vi "test -- PLL analyzer -- V2.vi"() -> ()   [LabVIEW 2017]
uses:
  lorentzian.ctl
  circle corners.ctl
  pid -- parameters.ctl
  <vilib>/event_ctls.llb/eventvkey.ctl
  cursor winow.ctl
  show-win- control.ctl
  PID action.ctl
  cursor window action.ctl
  agregator -- action.ctl
  interpolation state - real.ctl
  publisher action.ctl
  four-corner circle transformation.ctl
  cursor action.ctl
  linear interpolation - real.vi
  draw a line.vi
  draw a circle.vi
  linear interpolation iiii- complex.vi
  Q - not nan -- real.vi
  generate linear region.vi
panel:
  in  "all 3":enum32{"all", "other"}(tab)
  in  "reset freq":bool
  in  "dt (sec)":dbl=0.001 format="%#_10f"
  out "Plot: complex plane - filter":cluster{dbl[], dbl[]}[](graph)=[{[0.00032340920609960806, 0.00032267756333283855, 0.0003204839185825568, 0.0003168321202470601, 0.00031172857482151867, 0.00030518223565880506, 0.0002972045872622716, 0.0002878096251380292, 0.0002770138312420732, 0.00026483614506533264, 0.00025129793040736686, 0.00023642293789700238, 0.00022023726332565878, 0.00020276930186646325, 0.00018404969825946873, 0.00016411129305036554, 0.00014298906497700625, 0.00012072006960481285, 9.734337431872354e-05, 7.289998978572481e-05, 4.743279800820512e-05, 2.098647709435238e-05, -6.392577122430495e-06, -3.465633247758186e-05, -6.37552047401204e-05, -9.363814460023435e-05, -0.00012425272722711787, -0.0001555452442399381, -0.0001874607979305862, -0.00021994339757291058, -0.00025293605764947704, -0.00028638089782352986, -0.0003202192444807712, -0.00035439173366281644, -0.00038883841521175036, -0.00042349885794307543, -0.0004583122556625431, -0.0004932175338408814, -0.0005281534567592722, -0.0005630587349376105, -0.0005978721326570782, -0.000632532575388403, -0.0006669792569373372, -0.0007011517461193825, -0.0007349900927766238, -0.0007684349329506767, -0.0008014275930272432, -0.0008339101926695676, -0.0008658257463602154, -0.0008971182633730359, -0.0009277328459999193, -0.0009576157858600333, -0.000986714658122572, -0.0010149784134777233, -0.001042357467694506, -0.0010688037886083589, -0.0010942709803858784, -0.0011187143649188773, -0.0011420910602049665, -0.0011643600555771602, -0.0011854822836505194, -0.0012054206888596224, -0.0012241402924666172, -0.0012416082539258126, -0.0012577939284971562, -0.0012726689210075207, -0.0012862071356654864, -0.0012983848218422272, -0.0013091806157381832, -0.0013185755778624254, -0.001326553226258959, -0.0013330995654216725, -0.001338203110847214, -0.0013418549091827109, -0.0013440485539329924, -0.001344780196699762, -0.0013440485539329924, -0.0013418549091827109, -0.001338203110847214, -0.0013330995654216725, -0.001326553226258959, -0.0013185755778624257, -0.0013091806157381832, -0.0012983848218422272, -0.0012862071356654866, -0.001272668921007521, -0.0012577939284971564, -0.0012416082539258128, -0.0012241402924666174, -0.001205420688859623, -0.0011854822836505196, -0.0011643600555771604, -0.001142091060204967, -0.0011187143649188777, -0.0010942709803858789, -0.0010688037886083593, -0.0010423574676945067, -0.001014978413477724, -0.0009867146581225724, -0.0009576157858600338, -0.0009277328459999199, -0.0008971182633730364, -0.0008658257463602159, -0.0008339101926695678, -0.0008014275930272436, -0.000768434932950677, -0.000734990092776624, -0.0007011517461193834, -0.0006669792569373381, -0.000632532575388404, -0.000597872132657079, -0.0005630587349376113, -0.0005281534567592729, -0.000493217533840882, -0.0004583122556625437, -0.00042349885794307603, -0.0003888384152117509, -0.0003543917336628168, -0.00032021924448077157, -0.00028638089782353024, -0.0002529360576494772, -0.00021994339757291145, -0.00018746079793058703, -0.00015554524423993897, -0.00012425272722711857, -9.3638144600235e-05, -6.375520474012104e-05, -3.4656332477582454e-05, -6.392577122430929e-06, 2.0986477094351945e-05, 4.7432798008204685e-05, 7.289998978572449e-05, 9.734337431872332e-05, 0.00012072006960481252, 0.00014298906497700603, 0.00016411129305036543, 0.00018404969825946808, 0.00020276930186646292, 0.00022023726332565834, 0.00023642293789700205, 0.00025129793040736654, 0.0002648361450653323, 0.000277013831242073, 0.0002878096251380291, 0.0002972045872622715, 0.00030518223565880495, 0.00031172857482151856, 0.0003168321202470601, 0.0003204839185825567, 0.00032267756333283855], [0.00031496097830625033, 0.0003498892391994237, 0.00038475622405428764, 0.00041950076433152565, 0.00045406190630121736, 0.0004883790179763929, 0.0005223918954821412, 0.0005560408686736638, 0.0005892669058179846, 0.0006220117171556694, 0.0006542178571608702, 0.0006858288253202979, 0.0007167891652543217, 0.0007470445620063031, 0.0007765419373294864, 0.0008052295428042793, 0.0008330570506225647, 0.0008599756418797792, 0.0008859380922198584, 0.0009108988546828062, 0.0009348141396095384, 0.0009576419914638252, 0.000979342362436558, 0.0009998771827032147, 0.001019210427211269, 0.0010373081788803734, 0.0010541386881044424, 0.001069672428451252, 0.0010838821484618333, 0.0010967429194587922, 0.0011082321792796812, 0.0011183297718586971, 0.0011270179825872719, 0.0011342815693915135, 0.001140107789471984, 0.001144486421658899, 0.001147409784343534, 0.0011488727489543746, 0.0011488727489543746, 0.001147409784343534, 0.001144486421658899, 0.001140107789471984, 0.0011342815693915135, 0.001127017982587272, 0.0011183297718586971, 0.0011082321792796812, 0.0010967429194587925, 0.0010838821484618333, 0.0010696724284512522, 0.0010541386881044426, 0.0010373081788803734, 0.0010192104272112692, 0.0009998771827032147, 0.000979342362436558, 0.0009576419914638255, 0.0009348141396095387, 0.0009108988546828065, 0.0008859380922198587, 0.0008599756418797793, 0.000833057050622565, 0.0008052295428042794, 0.0007765419373294868, 0.0007470445620063036, 0.000716789165254322, 0.0006858288253202981, 0.0006542178571608704, 0.0006220117171556695, 0.0005892669058179848, 0.0005560408686736642, 0.0005223918954821417, 0.0004883790179763933, 0.00045406190630121763, 0.0004195007643315259, 0.00038475622405428786, 0.00034988923919942387, 0.0003149609783062508, 0.0002800327174130774, 0.0002451657325582134, 0.00021042119228097535, 0.00017586005031128358, 0.00014154293863610795, 0.00010753006113035959, 7.38810879388374e-05, 4.0655050794516443e-05, 7.910239456831666e-06, -2.429590054836919e-05, -5.590686870779693e-05, -8.68672086418208e-05, -0.00011712260539380236, -0.0001466199807169854, -0.00017530758619177826, -0.00020313509401006374, -0.00023005368526727817, -0.00025601613560735756, -0.00028097689807030546, -0.00030489218299703763, -0.0003277200348513243, -0.000349420405824057, -0.0003699552260907138, -0.0003892884705987683, -0.00040738622226787243, -0.0004242167314919416, -0.00043975047183875127, -0.00045396019184933253, -0.0004668209628462916, -0.0004783102226671804, -0.0004884078152461965, -0.0004970960259747711, -0.0005043596127790127, -0.0005101858328594831, -0.0005145644650463984, -0.0005174878277310334, -0.000518950792341874, -0.000518950792341874, -0.0005174878277310334, -0.0005145644650463984, -0.0005101858328594832, -0.0005043596127790129, -0.0004970960259747713, -0.0004884078152461966, -0.0004783102226671805, -0.000466820962846292, -0.00045396019184933286, -0.0004397504718387517, -0.00042421673149194215, -0.000407386222267873, -0.00038928847059876883, -0.00036995522609071434, -0.00034942040582405765, -0.00032772003485132494, -0.00030489218299703817, -0.0002809768980703059, -0.000256016135607358, -0.00023005368526727871, -0.0002031350940100644, -0.0001753075861917788, -0.00014661998071698658, -0.00011712260539380328, -8.686720864182172e-05, -5.590686870779785e-05, -2.429590054837011e-05, 7.910239456830636e-06, 4.065505079451547e-05, 7.388108793883637e-05, 0.00010753006113035894, 0.00014154293863610727, 0.00017586005031128293, 0.00021042119228097467, 0.00024516573255821275, 0.0002800327174130767]}, {[0.00017614197280843374, 0.00010745922599758267, 3.8776479186731605e-05, -2.990626762411946e-05, -9.858901443497053e-05, -0.00016727176124582157, -0.00023595450805667266, -0.00030463725486752375, -0.0003733200016783748, -0.00044200274848922583, -0.0005106854953000769, -0.000579368242110928, -0.000648050988921779, -0.0007167337357326301, -0.0007854164825434812, -0.0008540992293543323, -0.0009227819761651833, -0.0009914647229760344, -0.0010601474697868854, -0.0011288302165977364], [-0.00015830638794107768, -0.00011097965131634489, -6.365291469161208e-05, -1.6326178066879268e-05, 3.100055855785353e-05, 7.832729518258632e-05, 0.00012565403180731915, 0.00017298076843205192, 0.00022030750505678474, 0.00026763424168151756, 0.00031496097830625033, 0.0003622877149309831, 0.000409614451555716, 0.00045694118818044875, 0.0005042679248051815, 0.0005515946614299144, 0.0005989213980546472, 0.0006462481346793799, 0.0006935748713041128, 0.0007409016079288456]}, {[-0.000983952861547405, -0.0009366261249226722, -0.0008892993882979395, -0.0008419726516732066, -0.0007946459150484738, -0.000747319178423741, -0.0006999924417990082, -0.0006526657051742754, -0.0006053389685495426, -0.0005580122319248099, -0.0005106854953000771, -0.0004633587586753442, -0.00041603202205061144, -0.00036870528542587867, -0.0003213785488011458, -0.000274051812176413, -0.00022672507555168025, -0.00017939833892694748, -0.0001320716023022147, -8.474486567748183e-05], [-0.0003718664898022604, -0.00030318374299140934, -0.00023450099618055824, -0.00016581824936970718, -9.713550255885611e-05, -2.8452755748005075e-05, 4.022999106284602e-05, 0.00010891273787369711, 0.00017759548468454815, 0.0002462782314953992, 0.0003149609783062502, 0.00038364372511710137, 0.0004523264719279524, 0.0005210092187388034, 0.0005896919655496546, 0.0006583747123605056, 0.0007270574591713567, 0.0007957402059822077, 0.0008644229527930588, 0.0009331056996039098]}, {[-0.0007703927596862223, -0.0006757392864367567, -0.0005810858131872911, -0.00048643233993782547, -0.0003917788666883599, -0.0002971253934388943, -0.00020247192018942864, -0.0001078184469399631, -1.316497369049745e-05, 8.14884995589682e-05, 0.00017614197280843374, 0.0002707954460578993, 0.00036544891930736503, 0.00046010239255683057, 0.0005547558658062961, 0.0006494093390557619, 0.0007440628123052274, 0.0008387162855546929, 0.0009333697588041587, 0.0010280232320536242], [-0.001531961324158099, -0.001394595830536397, -0.0012572303369146947, -0.0011198648432929927, -0.0009824993496712906, -0.0008451338560495885, -0.0007077683624278863, -0.0005704028688061841, -0.00043303737518448206, -0.00029567188156278, -0.0001583063879410779, -2.0940894319375607e-05, 0.00011642459930232647, 0.00025379009292402855, 0.00039115558654573084, 0.0005285210801674329, 0.000665886573789135, 0.0008032520674108371, 0.0009406175610325391, 0.0010779830546542412]}]
  in  "PID parameters":T1={"P (sec)"=1.2701010101010102, "I (sec)"=0.7070707070707071}
  in  "visc hist time (sec)":dbl=15.0 format="%#_10f"
  in  "I (sec)":dbl(slide)=0.7070707070707071 scale=0.0..10.0
  in  "P (sec)":dbl(slide)=1.2701010101010102 scale=0.01..5.0
  in  "circle lorentzian":T2={"Amplitude"=0.002770252259498593, "omega(0)"=44853.30628564185, "Gamma"=3.3212682622846827, "phase"=4.109041090077058, "Q"=13504.87306158988, "Norm  Ampl"=nan, "z (inf)"=0.00017614197280843374-0.00015830638794107763i, "4corners"={"z (-pi/2)"=-0.0009839528615474048-0.0003718664898022611i, "z(inf)"=0.00017614197280843374-0.00015830638794107763i, "z (pi/2)"=-3.741812905274977e-05+0.001001788446414761i, "z center"=-0.0005106854953000773+0.00031496097830624995i, "z(0)"=-0.0011975129634085883+0.0007882283445535775i, "radius"=0.0008340947013996851}} {"z (inf)" format="%#9_9f"; "Q" format="%#9_9f"; "phase" format="%#9_9f"; "Gamma" format="%#9_9f"; "omega(0)" format="%#9_9f"}
  in  "time int ave time (sec)":dbl=0.05 format="%#_10f"
  in  "reset lor":bool
  in  "get fit!":bool
  in  "PLL away!":bool
  in  "PLL limits":dbl=5000.0 format="%#.2f"
  out "zi freq":dbl=44852.18508129662 format="%#.4f"
  out "off freq":dbl=1.1212043452251237 format="%#.8f"
  in  "cursor bracket: fit boundaries":T4={"left"=1.25, "right "=3.75, "center"=2.5, "window"=2.5, "cursors"=[0, 1, 2], "relative"=0, "absolute"=0, "fixed vertical offset"=0.0, "vertical offset"=0.0, "skew"=0.0, "default window frac"=0.1, "kind"=enum."symmetric", "skew.left"=0.5, "skew.right"=0.5, "Plot ref"=refnum, "wing order"=enum."forw"}
  out "VKey":T5
  out "Char":i16=49
  in  "lorentzian -- basic":T2={"Amplitude"=1.0, "omega(0)"=1000.0, "Gamma"=3.0, "phase"=0.0, "Q"=300.0, "Norm  Ampl"=nan, "z (inf)"=0.0+0.0i, "4corners"={"z (-pi/2)"=9.277908004825974e-07+0.0007240755403629966i, "z(inf)"=2.6527949823343002e-05+0.0007477540585896028i, "z (pi/2)"=2.8494315967368497e-06+0.0007733542176124632i, "z center"=1.8886111986097237e-06+0.0007487148789877299i, "z(0)"=-2.2750727426123552e-05+0.000749675699385857i, "radius"=2.4658065287076567e-05}} {"z (inf)" format="%#9_9f"; "Q" format="%#9_9f"; "phase" format="%#9_9f"; "Gamma" format="%#9_9f"; "omega(0)" format="%#9_9f"}
  out "DO reset freq !":bool
  in  "all":enum32{"all", "other"}(tab)
  in  "send for fit!":bool=TRUE
  out "Plot: complex- hist":cluster{dbl[], dbl[]}[](graph)
  out "Plot: hist":cluster{"all rows":dbl[], "all rows":dbl[]}[](graph)
  out "dev freq":dbl=44853.30628564185 format="%#.2f"
  out "win":T6={"center freq (Hz)"=-0.35260838541595674, "window  (Hz)"=17.234446484426172, "left freq (Hz)"=-8.969831627629043, "right freq (Hz)"=8.26461485679713}
  out "zi freq temporary":dbl=44852.18508134297 format="%#.2f"
  out "freq out":dbl[](array[numeric])
  out "v out":cdb[](array[numeric])
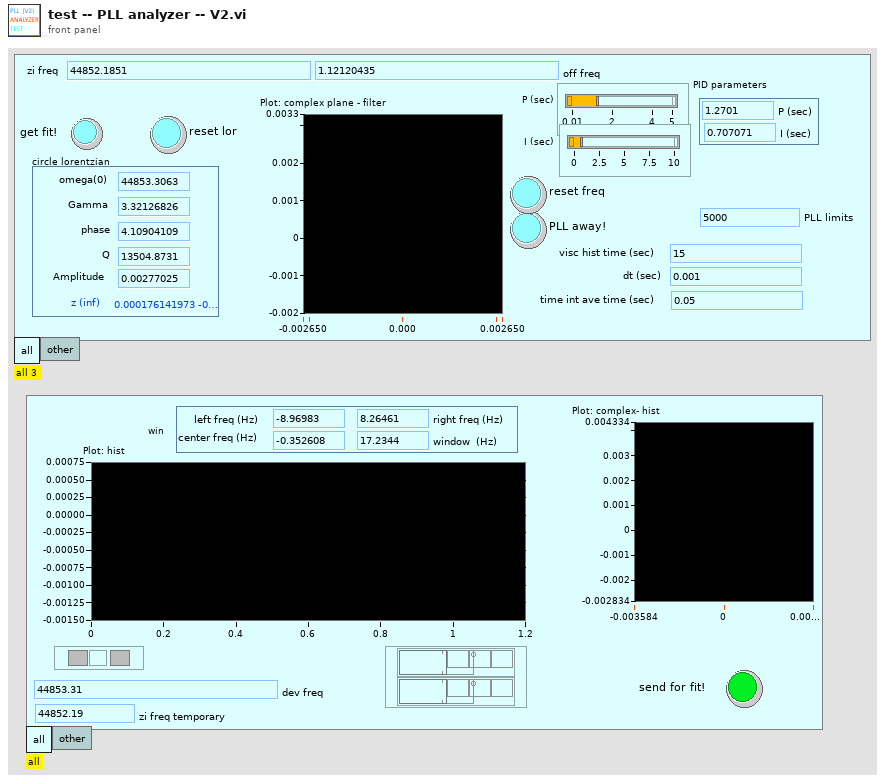
[diagram p1: front panel]
types:
  T1 = typedef "pid -- parameters.ctl" = cluster{"P (sec)":dbl, "I (sec)":dbl}
  T2 = typedef "lorentzian.ctl" = cluster{"Amplitude":dbl, "omega(0)":dbl, "Gamma":dbl, "phase":dbl, "Q":dbl, "Norm  Ampl":dbl, "z (inf)":cdb, "4corners":T3}
  T3 = typedef "circle corners.ctl" = cluster{"z (-pi/2)":cdb, "z(inf)":cdb, "z (pi/2)":cdb, "z center":cdb, "z(0)":cdb, "radius":dbl}
  T4 = typedef "cursor winow.ctl" = cluster{"left":dbl, "right ":dbl, "center":dbl, "window":dbl, "cursors":i32[], "relative":i32, "absolute":i32, "fixed vertical offset":dbl, "vertical offset":dbl, "skew":dbl, "default window frac":dbl, "kind":enum16{"symmetric", "skewed", "fancy"}, "skew.left":dbl, "skew.right":dbl, "Plot ref":refnum<vi>, "wing order":enum16{"forw", "back"}}
  T5 = typedef "eventvkey.ctl" = enum16{"ASCII", "Enter", "Return", "Shift", "Ctrl", "Alt", "Cmd", "Opt", "Caps", "NumLock", "Clear", "Break", "Up", "Down", "Left", "Right", "Insert", "Delete", "Home", "End", "PageUp", "PageDown", "Escape", "Help", "Pause", "ScrollLock", "F1", "F2", "F3", "F4", "F5", "F6", "F7", "F8", "F9", "F10", "F11", "F12", "F13", "F14", "F15", "F16", "F17", "F18", "F19", "F20", "F21", "F22", "F23", "F24", "Play", "VolumeUp", "VolumeDown", "Mute", "Two Byte Char"}
  T6 = typedef "show-win- control.ctl" = cluster{"center freq (Hz)":dbl, "window  (Hz)":dbl, "left freq (Hz)":dbl, "right freq (Hz)":dbl}
  T7 = typedef "publisher action.ctl" = enum16{"set", "get"}
  T8 = typedef "interpolation state - real.ctl" = cluster{"requested size":i32, "Array":dbl[], "actual number of elements":i32}
  T9 = typedef "agregator -- action.ctl" = enum16{"append", "interpolate", "empty!", "force", "init", "scale", "read last"}
  T10 = typedef "cursor window action.ctl" = enum16{"balance", "h. offset change", "cursor moves", "change center", "change window", "init", "check", "reset", "set y to middle", "idle", "-write all Y", "-write left.X", "-write center.X", "-write right.X", "-write all X", "-change center", "-change window", "-change skew", "-read cursor 2", "-read cursor 1", "-read cursor 0", "-read all cursors", "-reset", "-read plot scale", "-set y to middle", "-Q: center.Y is visible", "-Q: window is visible", "-parse center.Y", "-right left from center", "-left move", "-right move", "-set center.Y", "-empty", "-set cursors to default", "-check", "-write center.Y", "-copy cursor 1", "-copy cursor 0", "-copy cursor 2", "move right", "move left", "shrink", "broaden", "skew up", "skew down", "-write plot scale", "zoom X", "change cen&win", "zoom to all data", "color--red", "color--green", "color--yellow", "read", "zoom out", "zoom in", "slide right", "slide left", "set range aspect ratio to 1"}
  T11 = typedef "PID action.ctl" = enum16{"append", "empty!", "reset frequency"}
  T12 = typedef "Zurich Instruments LabOne.lvlib/ziTypeHandle.ctl" = cluster{"handleValid":bool, "Conn":u64, "Path Prefix":string, "Handle":u64, "Connected":bool, "Clockbase(s)":dbl}
  T13 = typedef "cursor action.ctl" = enum16{"range", "read", "write", "check", "zoom out", "smart zoom out", "zoom to aspect ratio 1"}
  T14 = typedef "four-corner circle transformation.ctl" = enum16{"z(c) z(inf)", "z(c) z(zero)", "fix phase", "calculate lorentzian", "z(0) z(+-pi/2)", "shift to zcenter", "to  canonical", "get canonical phase", "get4corners"}
  T15 = typedef "interpolation state - complex.ctl" = cluster{"requested size":i32, "Array":cdb[], "actual number of elements":i32}
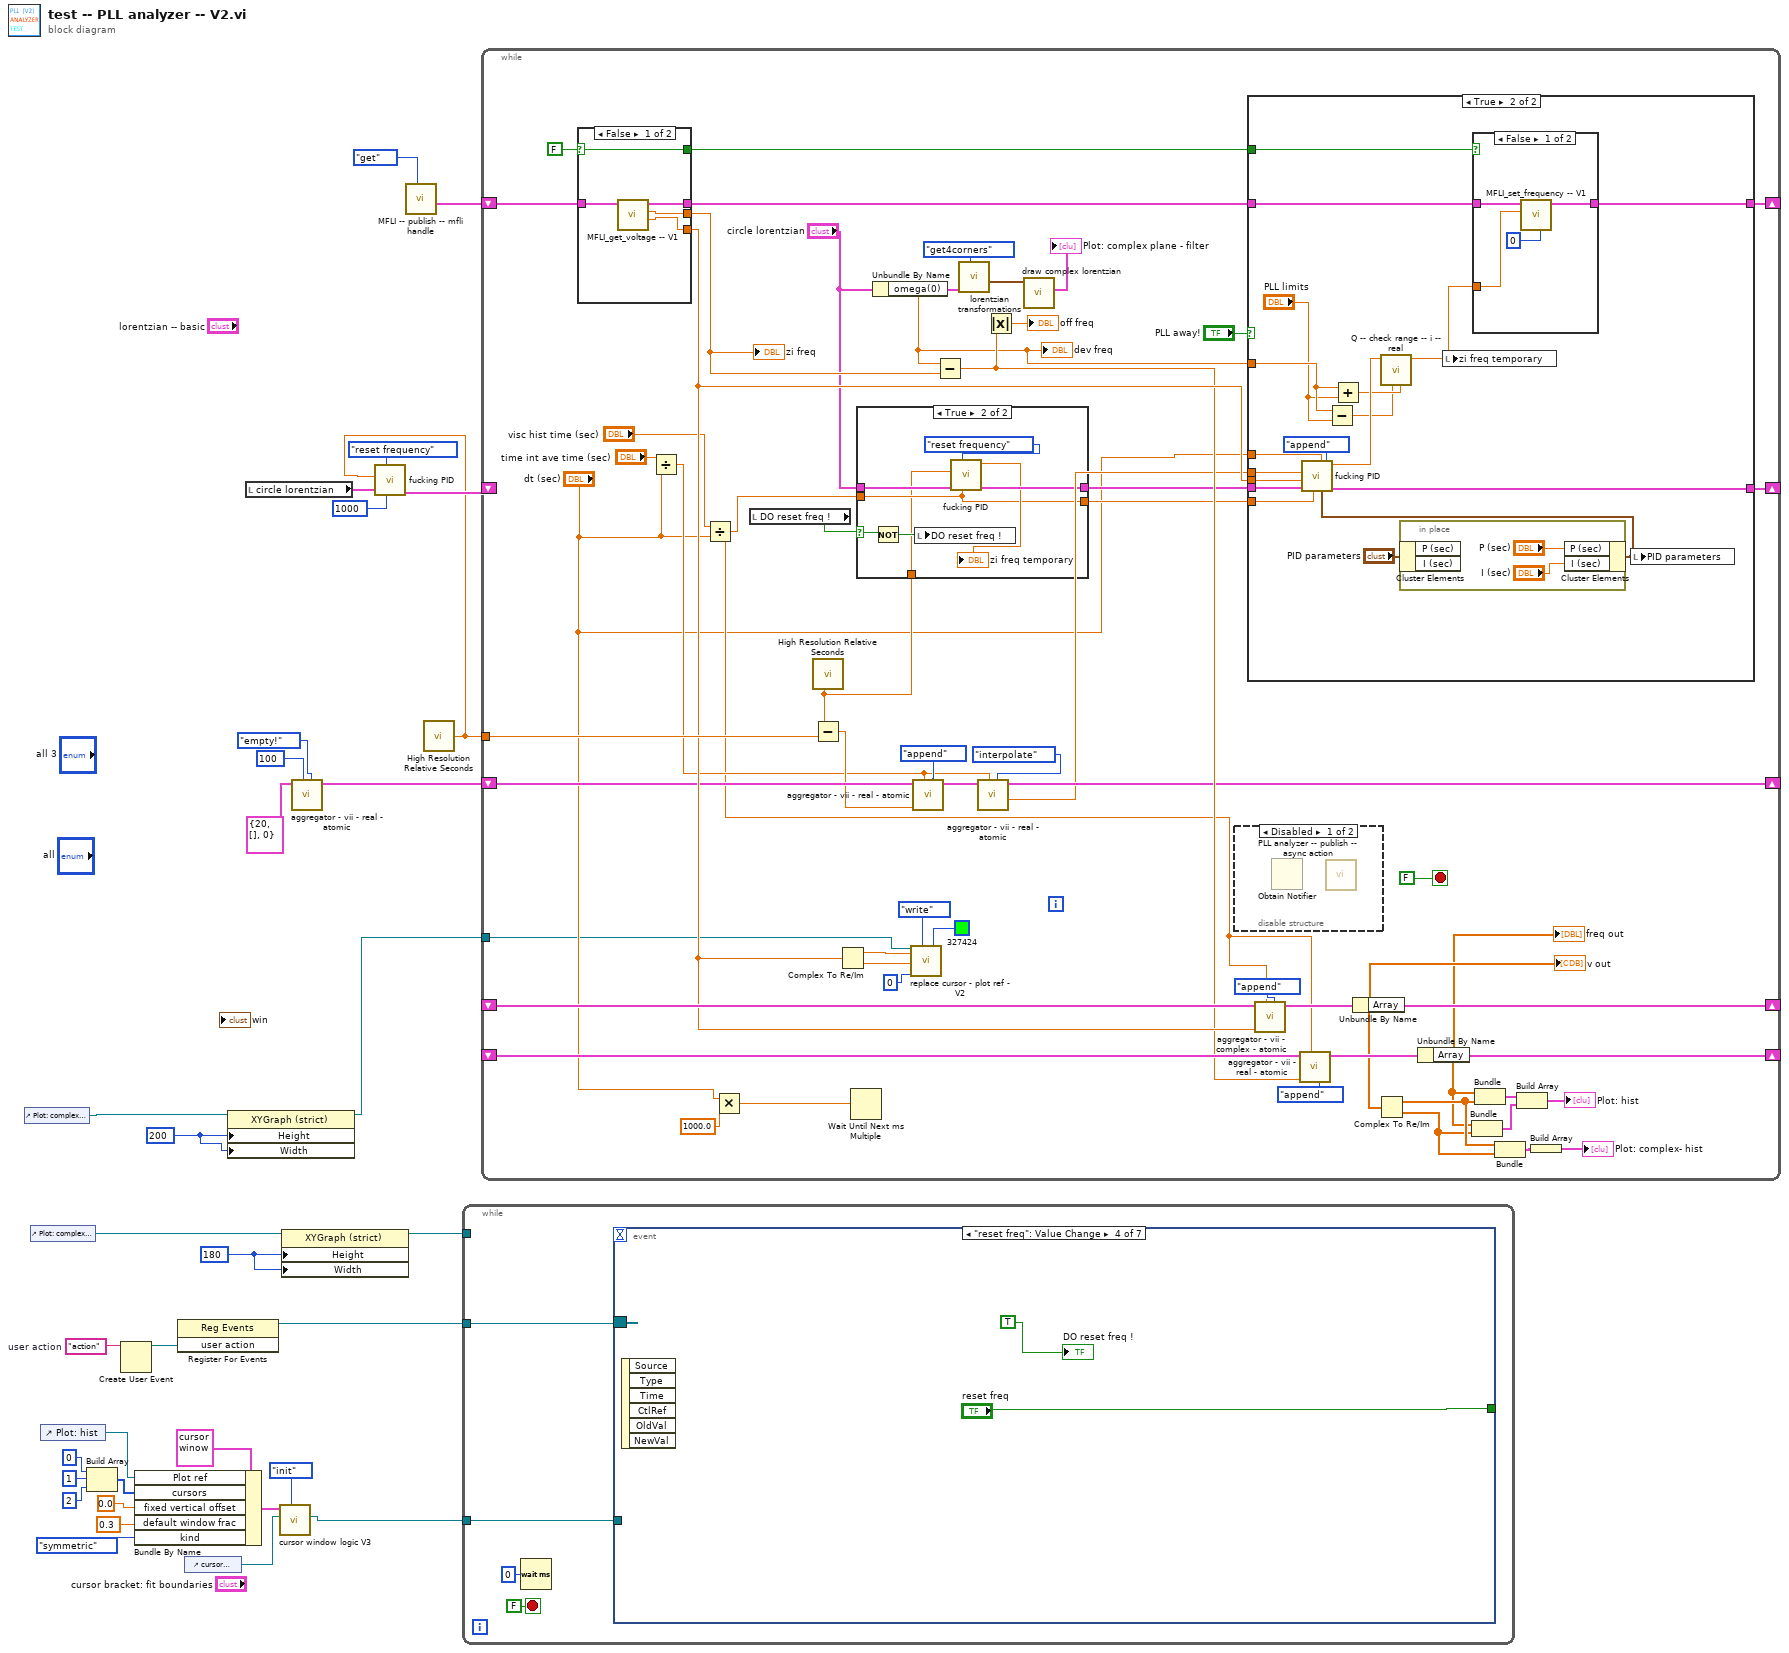
[diagram p0: block diagram]
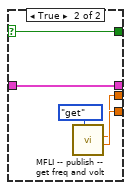
[diagram p2: hidden frame]
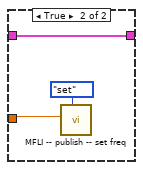
[diagram p4: hidden frame]
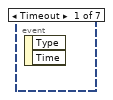
[diagram p7: hidden frame]
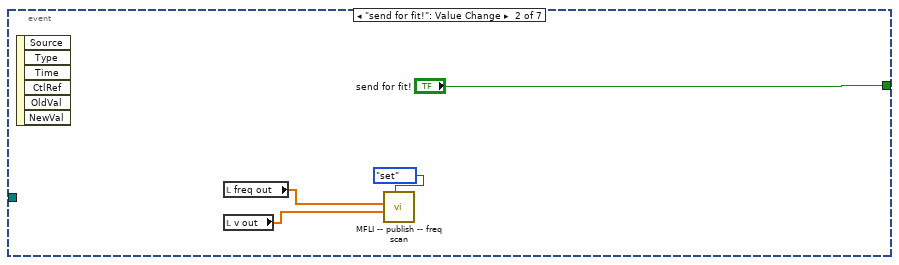
[diagram p8: hidden frame]
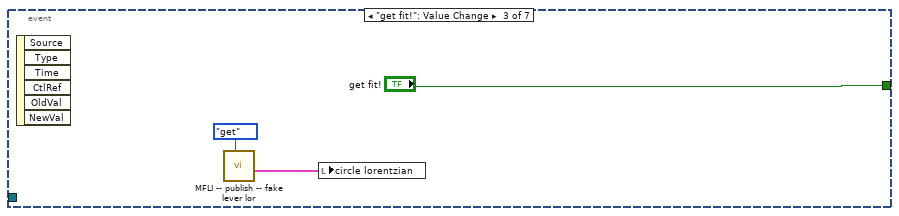
[diagram p9: hidden frame]
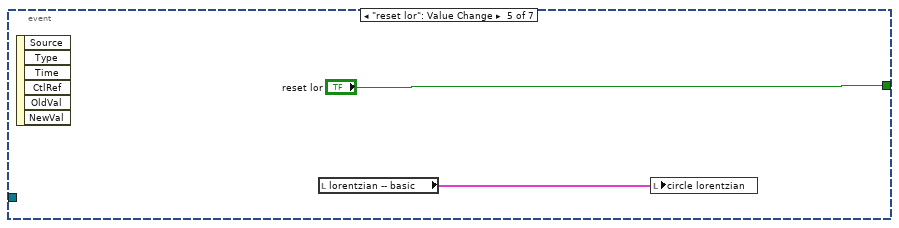
[diagram p10: hidden frame]
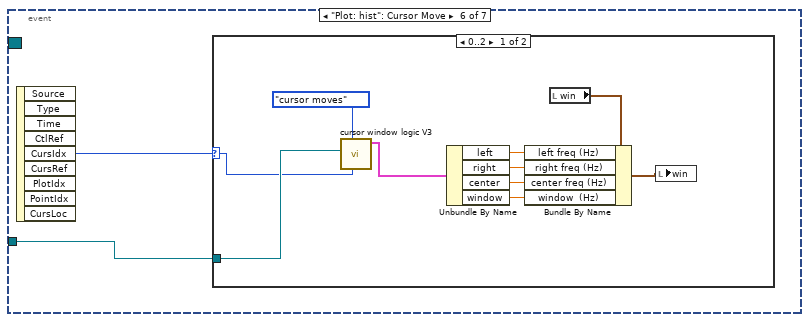
[diagram p11: hidden frame]
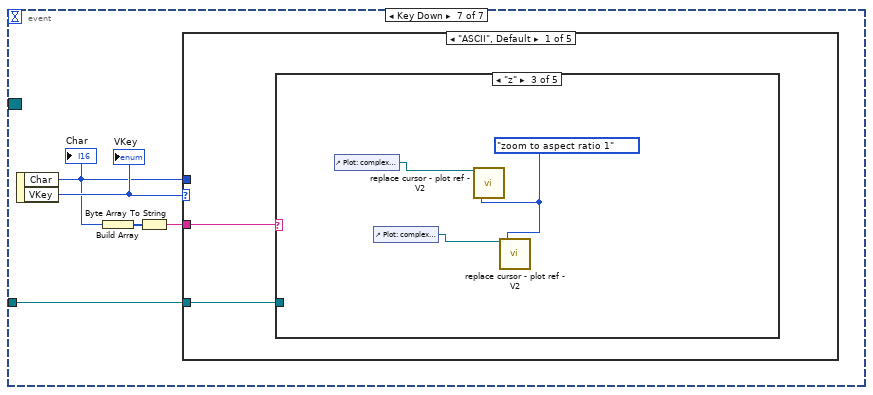
[diagram p13: hidden frame]
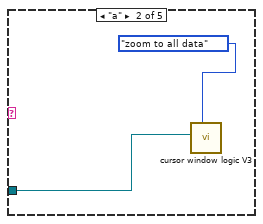
[diagram p15: hidden frame]
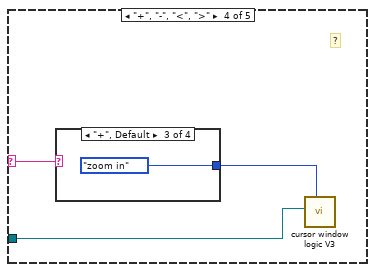
[diagram p16: hidden frame]
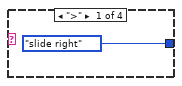
[diagram p17: hidden frame]
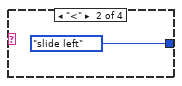
[diagram p18: hidden frame]
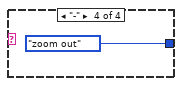
[diagram p19: hidden frame]
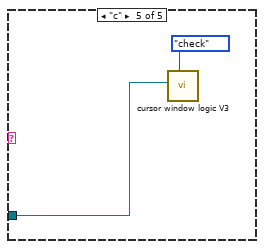
[diagram p20: hidden frame]
diagram:
  w4 = u32 180 ("Plot Area:Size:Height")
  w6 = u32 200 ("Plot Area:Size:Height")
  w30 = "action"  # user action
  n1 = control-ref of="Plot: complex plane - filter"() -> (w7:refnum<vi>)
  n2 = control-ref of="Plot: complex- hist"() -> (w1:refnum<vi>)
  n3 = control-ref of="Plot: hist"() -> (w3:refnum<vi>)
  n4 = Build Array(0, 1, 2) -> (w18:i32[])
  n5 = Create User Event(user event datatype=w30) -> (user event=w31:refnum<user-event>)  [unwired: 1 in, 1 out]
  n6 = Bundle By Name(cluster=T4 {"left"=0.0, "right "=0.0, "center"=0.0, "window"=0.0, "cursors"=[], "relative"=0, "absolute"=0, "fixed vertical offset"=0.0, "vertical offset"=0.0, "skew"=0.0, "default window frac"=0.0, "kind"=enum."symmetric", "skew.left"=0.0, "skew.right"=0.0, "Plot ref"=refnum, "wing order"=enum."forw"} ("cursor bracket: All, data window"), "Plot ref"=w3, "cursors"=w18, "fixed vertical offset"=0.0, "default window frac"=0.3 ("fixed vertical offset"), "kind"=enum16{"symmetric", "skewed", "fancy"}."symmetric") -> (w26:T4)
  n7 = register-events(w31) -> (reference out=w29:refnum<event-registration>)  [unwired: 2 in, 1 out]
  n8 = control-ref of="cursor bracket: fit boundaries"() -> (w28:refnum<vi>)
  n9 = property class="XYGraph (strict)"(reference=w7, "Height"=w6, "Width"=w6) -> (reference out=w5:refnum<vi>)  [unwired: 1 in, 1 out]
  n10 = local read "circle lorentzian"() -> (w14:T2)
  n11 = call "cursor window logic V3.vi"("cursor window action"=cursor_window_action."init", "cursor window in"=w28, "cursor window init"=w26) -> ("cursor window out"=w32:refnum<vi>)  [unwired: 7 in, 1 out]
  n12 = property class="XYGraph (strict)"(reference=w1, "Height"=w4, "Width"=w4) -> (reference out=w2:refnum<vi>)  [unwired: 1 in, 1 out]
  n13 = call "aggregator - vii - real - atomic.vi"("aggregator action"=agregator_--_action."empty!", "requested size"=100, "state IN"=T8 {"requested size"=20, "Array"=[], "actual number of elements"=0}) -> ("state OUT"=w17:T8)  [unwired: 5 in, 3 out]
  n14 = call "MFLI -- publish -- mfli handle.vi"("publisher action"=publisher_action."get") -> ("Handle Out"=w12:T12)  [unwired: 10 in]
  n15 = call <vilib>:"High Resolution Relative Seconds.vi"() -> ("relative seconds"=w8:dbl)
  n16 = call "fucking PID.vi"("requested size"=1000, "PID action"=PID_action."reset frequency", "lorentzian IN"=w14, "time in (sec)"=w8) -> ("lorentzian  OUT"=w11:T2)  [unwired: 4 in, 3 out]
  n17 = while {
    tunnel: w29 -> [w37]
    tunnel: w32 -> [w35]
    tunnel: w2 -> [_]
    stop <- FALSE stop-if-true
    n18 = Wait (ms)(milliseconds to wait=u32 0) -> ()  [unwired: 1 out]
    n19 = event shown="[3] \"reset freq\": Value Change" {
      selector: w37 -> [_ _ _ _ _ _ _]
      dyn-events: _ -> [_ _ _ _ _ _ _]
      timeout: _ -> [_ _ _ _ _ _ _]
      tunnel: w35 -> [_ _ _ _ _ w50 w61]
      tunnel: [_ "send for fit!" "get fit!" "reset freq" "reset lor" _ _] -> _
      event Timeout {
        n20 = event-data() -> ()  [unwired: 1 in, 2 out]
      }
      event "send for fit!": Value Change {
        n21 = event-data() -> ()  [unwired: 1 in, 6 out]
        n22 = local read "freq out"() -> (w40:dbl[])
        n23 = local read "v out"() -> (w39:cdb[])
        n24 = call "MFLI -- publish -- freq scan.vi"("publisher action"=publisher_action."set", "Voltage IN (V)"=w39, "Freq IN (Hz)"=w40) -> ()  [unwired: 7 in, 2 out]
      }
      event "get fit!": Value Change {
        n25 = event-data() -> ()  [unwired: 1 in, 6 out]
        n26 = call "MFLI -- publish -- fake lever lor.vi"("publisher action"=publisher_action."get") -> ("lorentzian OUT"=w42:T2)  [unwired: 10 in]
        n27 = local write "circle lorentzian"(w42) -> ()
      }
      event "reset freq": Value Change {
        n28 = event-data() -> ()  [unwired: 1 in, 6 out]
        "DO reset freq !" <- TRUE ("DO reset freq !")
      }
      event "reset lor": Value Change {
        n29 = event-data() -> ()  [unwired: 1 in, 6 out]
        n30 = local read "lorentzian -- basic"() -> (w47:T2)
        n31 = local write "circle lorentzian"(w47) -> ()
      }
      event "Plot: hist": Cursor Move {
        n32 = event-data() -> ("CursIdx"=w49:i32)  [unwired: 1 in, 8 out]
        n33 = case shown="0..2" w49 {
          selector: w49 -> [w58 _]
          tunnel: w50 -> [w60 _]
          frame 0..2 {
            n34 = call "cursor window logic V3.vi"("CursIdx"=w58, "cursor window action"=cursor_window_action."cursor moves", "cursor window in"=w60) -> ("cursor window out"=w57:T4)  [unwired: 7 in, 1 out]
            n35 = Unbundle By Name(w57) -> ("left"=w55:dbl, "right"=w54:dbl, "center"=w53:dbl, "window"=w52:dbl)
            n36 = local read "win"() -> (w56:T6)
            n37 = Bundle By Name(cluster=w56, "left freq (Hz)"=w55, "right freq (Hz)"=w54, "center freq (Hz)"=w53, "window  (Hz)"=w52) -> (w51:T6)
            n38 = local write "win"(w51) -> ()
          }
          frame 3, Default {
          }
        }
      }
      event Key Down {
        n39 = event-data() -> ("Char"=w63:i16, "VKey"=w65:T5)  [unwired: 1 in]
        "Char" <- w63
        "VKey" <- w65
        n40 = Build Array(w63) -> (w64:i16[])
        n41 = Byte Array To String(unsigned byte array=w64) -> (string=w62:string)
        n42 = case shown="\"ASCII\", Default" w65 {
          selector: w65 -> [_ _ _ _ w91]
          tunnel: w63 -> [_ _ _ _ _]
          tunnel: w62 -> [w67 _ _ _ _]
          tunnel: w61 -> [w66 _ _ _ w89]
          frame "ASCII", Default {
            n43 = case shown="\"z\"" w67 {
              selector: w67 -> [_ _ _ w74 _]
              tunnel: w66 -> [_ w68 _ w75 w80]
              frame "0", Default {
              }
              frame "a" {
                n44 = call "cursor window logic V3.vi"("cursor window action"=cursor_window_action."zoom to all data", "cursor window in"=w68) -> ()  [unwired: 8 in, 2 out]
              }
              frame "z" {
                w71 = cursor_action."zoom to aspect ratio 1" ("cursor action")
                n45 = control-ref of="Plot: complex plane - filter"() -> (w72:refnum<vi>)
                n46 = control-ref of="Plot: complex- hist"() -> (w70:refnum<vi>)
                n47 = call "replace cursor - plot ref - V2.vi"("Plot ref in"=w72, "cursor action"=w71) -> ()  [unwired: 15 in, 3 out]
                n48 = call "replace cursor - plot ref - V2.vi"("Plot ref in"=w70, "cursor action"=w71) -> ()  [unwired: 15 in, 3 out]
              }
              frame "+", "-", "<", ">" {
                # "?"
                n49 = case shown="\"+\", Default" w74 {
                  tunnel: [cursor_window_action."slide right" ("cursor window action") cursor_window_action."slide left" ("cursor window action") cursor_window_action."zoom in" ("cursor window action") cursor_window_action."zoom out" ("cursor window action")] -> w73
                  frame ">" {
                  }
                  frame "<" {
                  }
                  frame "+", Default {
                  }
                  frame "-" {
                  }
                }
                n50 = call "cursor window logic V3.vi"("cursor window action"=w73, "cursor window in"=w75) -> ()  [unwired: 8 in, 2 out]
              }
              frame "c" {
                n51 = call "cursor window logic V3.vi"("cursor window action"=cursor_window_action."check", "cursor window in"=w80) -> ()  [unwired: 8 in, 2 out]
              }
            }
          }
          frame "Escape" {
          }
          frame "PageUp" {
          }
          frame "PageDown" {
          }
          frame "Up".."Right" {
            n52 = case shown="\"Left\"" w91 {
              tunnel: [cursor_window_action."move right" ("cursor window action") cursor_window_action."move left" ("cursor window action") cursor_window_action."broaden" ("cursor window action") cursor_window_action."shrink" ("cursor window action")] -> w90
              frame "Right", Default {
              }
              frame "Left" {
              }
              frame "Up" {
              }
              frame "Down" {
              }
            }
            n53 = call "cursor window logic V3.vi"("cursor window action"=w90, "cursor window in"=w89) -> ("cursor window out"=w82:T4)  [unwired: 8 in, 1 out]
            n54 = Unbundle By Name(w82) -> ("left"=w84:dbl, "right"=w85:dbl, "center"=w86:dbl, "window"=w87:dbl)
            n55 = local read "win"() -> (w83:T6)
            n56 = Bundle By Name(cluster=w83, "left freq (Hz)"=w84, "right freq (Hz)"=w85, "center freq (Hz)"=w86, "window  (Hz)"=w87) -> (w88:T6)
            n57 = local write "win"(w88) -> ()
          }
        }
      }
    }
  }
  n58 = while {
    tunnel: w8 -> [w152]
    shift-right: [w143] -> _
    shift-left: w11 -> [_]
    shift-right: [w133] -> _
    shift-left: _ -> [w139]
    shift-right: [w134] -> _
    shift-left: _ -> [w136]
    shift-right: [w120] -> _
    shift-left: w17 -> [w123]
    shift-right: [w109] -> _
    shift-left: w12 -> [w107]
    tunnel: w5 -> [w96]
    stop <- FALSE stop-if-true
    n59 = case shown="False" FALSE {
      selector: FALSE -> [w157 w158]
      tunnel: [w153 w161] -> w131
      tunnel: [w154 w160] -> w130
      tunnel: [w155 w159] -> w108
      tunnel: w107 -> [w156 w159]
      tunnel: [w157 w158] -> w106
      frame False {
        n60 = call "MFLI_get_voltage -- V1.vi"("Handle In"=w156) -> ("z out (V)"=w153:cdb, "Freq out (Hz)"=w154:dbl, "Handle Out"=w155:T12)  [unwired: 7 in, 1 out]
      }
      frame True {
        n61 = call "MFLI -- publish -- get freq and volt.vi"("publisher action"=publisher_action."get") -> ("Voltage out (V)"=w161:cdb, "freq out (Hz)"=w160:dbl)  [unwired: 9 in]
      }
    }
    "zi freq" <- w130
    n62 = Divide(x="time int ave time (sec)", y="dt (sec)") -> (x/y=w102:dbl)
    n63 = Divide(x="visc hist time (sec)", y="dt (sec)") -> (x/y=w100:dbl)
    n64 = Multiply(x="dt (sec)", y=1000.0) -> (x*y=w115:dbl)
    n65 = local read "DO reset freq !"() -> (w114:bool)
    n66 = call <vilib>:"High Resolution Relative Seconds.vi"() -> ("relative seconds"=w98:dbl)
    n67 = Subtract(x=w98, y=w152) -> (x-y=w122:dbl)
    n68 = Complex To Re/Im(x + iy=w131) -> (x=w145:dbl, y=w144:dbl)
    n69 = Wait Until Next ms Multiple(millisecond multiple=w115) -> ()  [unwired: 1 out]
    n70 = case shown="True" w114 {
      selector: w114 -> [_ w198]
      tunnel: "circle lorentzian" -> [w193 w200]
      tunnel: [w193 w199] -> w112
      tunnel: w100 -> [w192 w195]
      tunnel: [w192 w195] -> w99
      tunnel: w98 -> [_ w194]
      frame False {
      }
      frame True {
        n71 = Not(x=w198) -> (.not. x?=w197:bool)
        n72 = local write "DO reset freq !"(w197) -> ()
        n73 = call "fucking PID.vi"("requested size"=w195, "PID action"=PID_action."reset frequency", "lorentzian IN"=w200, "time in (sec)"=w194) -> ("lorentzian  OUT"=w199:T2, "frequency out (Hz)"=→"zi freq temporary":dbl)  [unwired: 4 in, 2 out]
      }
    }
    n74 = Unbundle By Name("circle lorentzian") -> ("omega(0)"=w101:dbl)
    "dev freq" <- w101
    n75 = call "replace cursor - plot ref - V2.vi"("Plot ref in"=w96, "new X"=w145, "new  Y"=w144, "cursor index"=0, "cursor action"=cursor_action."write", "Color Box"=u32 327424) -> ()  [unwired: 11 in, 3 out]
    n76 = call "aggregator - vii - real - atomic.vi"("aggregator action"=agregator_--_action."append", "requested size"=w102, "number"=w122, "state IN"=w123) -> ("state OUT"=w121:T8)  [unwired: 4 in, 3 out]
    n77 = Subtract(x=w101, y=w130) -> (x-y=w129:dbl)
    n78 = call "lorentzian transformations.vi"("4 corner circle transformation"=four-corner_circle_transformation."get4corners", "lorentzian in"="circle lorentzian") -> ("4corners our"=w150:T3)  [unwired: 7 in, 2 out]
    n79 = call "aggregator - vii - real - atomic.vi"("aggregator action"=agregator_--_action."interpolate", "requested size"=w102, "state IN"=w121) -> ("interp average"=w118:dbl, "state OUT"=w120:T8)  [unwired: 5 in, 2 out]
    n80 = Absolute Value(x=w129) -> (abs(x)=→"off freq":dbl)
    n81 = call "draw complex lorentzian.vi"("4 corners"=w150) -> ("fancy circles"=→"Plot: complex plane - filter":cluster{dbl[], dbl[]}[])  [unwired: 10 in]
    n82 = disable-structure shown="Disabled" {
      frame Disabled {
        n83 = Obtain Notifier() -> ()  [unwired: 4 in, 3 out]
        n84 = call "PLL analyzer -- publish -- async action.vi"() -> ()  [unwired: 11 in, 1 out]
      }
      frame Enabled {
      }
    }
    n85 = case shown="True" "PLL away!" {
      tunnel: [w164 w182] -> w143
      tunnel: w99 -> [_ w180]
      tunnel: w131 -> [_ w177]
      tunnel: w118 -> [_ w176]
      tunnel: w112 -> [w164 w175]
      tunnel: [w163 w174] -> w109
      tunnel: w108 -> [w163 w173]
      tunnel: w106 -> [_ w172]
      tunnel: w101 -> [_ w169]
      tunnel: "dt (sec)" -> [_ w165]
      frame False {
      }
      frame True {
        n86 = Subtract(x=w169, y="PLL limits") -> (x-y=w167:dbl)
        n87 = Add(x=w169, y="PLL limits") -> (x+y=w170:dbl)
        n88 = in-place {
          n89 = in-place-cluster #1("PID parameters") -> ()  [unwired: 2 out]
          n90 = in-place-cluster #1("P (sec)"="P (sec)", "I (sec)"="I (sec)") -> (w178:T1)
        }
        n91 = call "fucking PID.vi"("PID parameters"=w178, "dt (sec)"=w165, "requested size"=w180, "PID action"=PID_action."append", "lorentzian IN"=w175, "voltage IN (V)"=w177, "time in (sec)"=w176) -> ("lorentzian  OUT"=w182:T2, "frequency out (Hz)"=w171:dbl)  [unwired: 1 in, 2 out]
        n92 = call "Q -- check range -- i -- real.vi"("upper"=w170, "lower"=w167, "number"=w171) -> ("number in range"=w166:dbl)  [unwired: 6 in, 2 out]
        n93 = local write "zi freq temporary"(w166) -> ()
        n94 = case shown="False" w172 {
          tunnel: w166 -> [w183 w188]
          tunnel: [w185 w187] -> w174
          tunnel: w173 -> [w186 w187]
          frame False {
            n95 = call "MFLI_set_frequency -- V1.vi"("Oscillator (0)"=u16 0, "Freq in (Hz)"=w183, "Handle In"=w186) -> ("Handle Out"=w185:T12)  [unwired: 5 in, 3 out]
          }
          frame True {
            n96 = call "MFLI -- publish -- set freq.vi"("publisher action"=publisher_action."set", "freq IN (Hz)"=w188) -> ()  [unwired: 9 in, 1 out]
          }
        }
        n97 = local write "PID parameters"(w178) -> ()
      }
    }
    n98 = call "aggregator - vii - complex - atomic.vi"("aggregator action"=agregator_--_action."append", "requested size"=w100, "number"=w131, "state IN"=w139) -> ("state OUT"=w133:T15)  [unwired: 4 in, 3 out]
    n99 = call "aggregator - vii - real - atomic.vi"("aggregator action"=agregator_--_action."append", "requested size"=w100, "number"=w129, "state IN"=w136) -> ("state OUT"=w134:T8)  [unwired: 4 in, 3 out]
    n100 = Unbundle By Name(w133) -> ("Array"=w132:cdb[])
    "v out" <- w132
    n101 = Complex To Re/Im(x + iy=w132) -> (x=w127:dbl[], y=w126:dbl[])
    n102 = Unbundle By Name(w134) -> ("Array"=w116:dbl[])
    "freq out" <- w116
    n103 = Bundle("Array"=w116, w126) -> (w141:cluster{"Array":dbl[], dbl[]})  [unwired: 1 in]
    n104 = Bundle("Array"=w116, w127) -> (w142:cluster{"Array":dbl[], dbl[]})  [unwired: 1 in]
    n105 = Bundle(w127, w126) -> (w128:cluster{dbl[], dbl[]})  [unwired: 1 in]
    n106 = Build Array(w142, w141) -> (→"Plot: hist":cluster{"Array":dbl[], dbl[]}[])
    n107 = Build Array(w128) -> (→"Plot: complex- hist":cluster{dbl[], dbl[]}[])
  }
